vi "wait_for_T.vi"(9 "Toleranz (%)":dbl, 10 "VISA session 2":refnum<visa-resource-name>, 11 "T_target":dbl) -> (2 "dup VISA session":refnum<visa-resource-name>, 3 "T innerhalb Toleranz":bool)   [LabVIEW 2010]
uses:
  Data_Display_global.vi
  Instrument_Setup.vi
  Programme/National Instruments/LabVIEW 8.5/instr.lib/Mischerinstr.lib/AVS-Brücke/LV Drivers for AVS/AVS47IB.LLB/AVS47IB Wait for OPC/MAV/TMO.vi
panel:
  in  "Delay (sec)":i16=1 min=0 max=3600 step=1
  in  "iter":i32=50
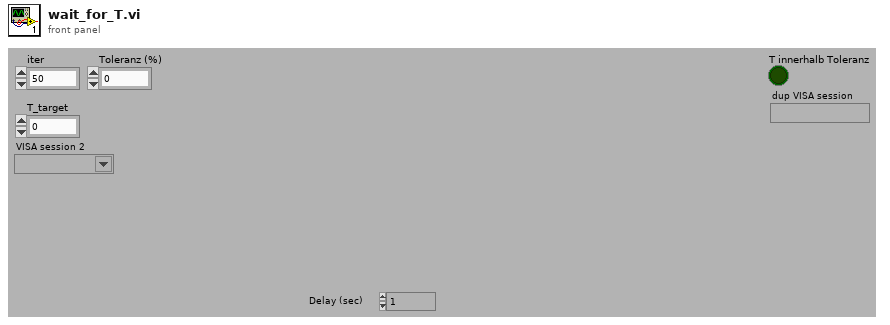
[diagram p1: front panel]
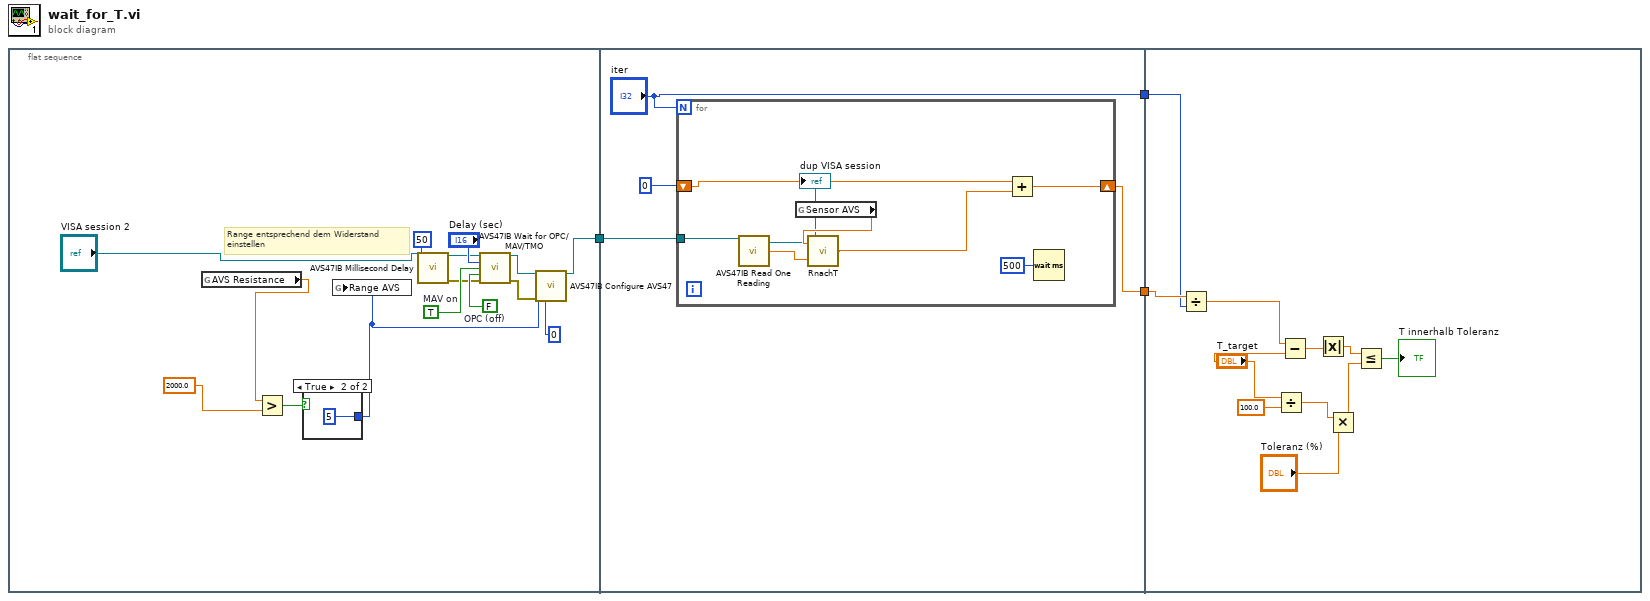
[diagram p0: block diagram]
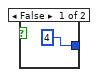
[diagram p2: hidden frame]
diagram:
  n1 = flat-sequence {
    tunnel: [w8] -> w1
    tunnel: [w23] -> w3
    tunnel: ["iter"] -> w2
    tunnel: w1 -> [w21]
    tunnel: w3 -> [w43]
    tunnel: w2 -> [w42]
    frame #0 {
      w17 = FALSE  # OPC (off)
      w18 = TRUE  # MAV on
      # "Range entsprechend dem Widerstand\neinstellen"
      n2 = global read "Data_Display_global.vi" "AVS Resistance"() -> (w4:dbl)
      n3 = Greater?(x=w4, y=2000.0) -> (0:w7:bool)
      n4 = case shown="True" w7 {
        tunnel: [i8 4 ("DISPLAY (-1:no change)") i8 5 ("DISPLAY (-1:no change)")] -> w5
        frame False {
        }
        frame True {
        }
      }
      n5 = global write "Instrument_Setup.vi" "Range AVS"(w5) -> ()
      n6 = call "AVS47IB Millisecond Delay.vi"("VISA session"="VISA session 2", "Delay (50 ms)"=50) -> ("dup VISA session"=w15:refnum<visa-resource-name>, "error out"=w14:errorcluster)  [unwired: 12 in]
      n7 = call "AVS47IB Wait for OPC/MAV/TMO.vi"("VISA session"=w15, "Timeout (2 sec)"="Delay (sec)", "MAV (on)"=w18, "OPC (off)"=w17, "error in (no error)"=w14) -> ("dup VISA session"=w12:refnum<visa-resource-name>, "error out"=w11:errorcluster)  [unwired: 8 in, 1 out]
      n8 = call "AVS47IB Configure AVS47.vi"("VISA session"=w12, "RANGE  (-1:no change)"=w5, "error in (no error)"=w11, "DISPLAY (-1:no change)"=i8 0) -> ("dup VISA session"=w8:refnum<visa-resource-name>)  [unwired: 10 in, 1 out]
    }
    frame #1 {
      n9 = for {
        N: "iter" -> [_]
        shift-right: [w31] -> w23
        shift-left: 0 -> [w32]
        tunnel: w21 -> [w25]
        n10 = call "AVS47IB Read One Reading.vi"("VISA session"=w25) -> ("dup VISA session"=→"dup VISA session":refnum<visa-resource-name>, "Resistance reading"=w29:dbl)  [unwired: 10 in, 3 out]
        n11 = global read "Instrument_Setup.vi" "Sensor AVS"() -> (w30:dbl)
        n12 = call "RnachT.vi"("R"=w29, "Sensor Cal #"=w30) -> ("T (K)"=w27:dbl)
        n13 = Add(x=w32, y=w27) -> (x+y=w31:dbl)
        n14 = Wait (ms)(milliseconds to wait=u32 500) -> ()  [unwired: 1 out]
      }
    }
    frame #2 {
      n15 = Divide(x=w43, y=w42) -> (x/y=w41:dbl)
      n16 = Divide(x="T_target", y=100.0) -> (x/y=w37:dbl)
      n17 = Subtract(x=w41, y="T_target") -> (x-y=w34:dbl)
      n18 = Absolute Value(x=w34) -> (abs(x)=w33:dbl)
      n19 = Multiply(x=w37, y="Toleranz (%)") -> (x*y=w35:dbl)
      n20 = Less Or Equal?(x=w33, y=w35) -> (x <= y?=→"T innerhalb Toleranz":bool)
    }
  }
